vi "Read_LCR_Meter_4192A.vi"() -> ()   [LabVIEW 2018]
panel:
  in  "GPIB addess":string="0:17"
  out "display B":dbl=20.0 format="%.3e"
  out "display A":dbl=0.02 format="%.3e"
  in  "Freq Value (Hz) (25Hz)":dbl=25.0
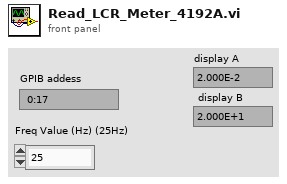
[diagram p1: front panel]
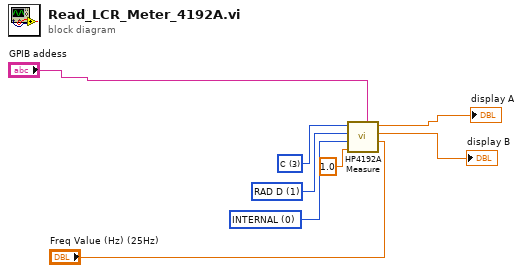
[diagram p0: block diagram]
diagram:
  w2 = i16 1 items=["DEG Q", "RAD D", "         R/G"] ("function B (deg q:0)")
  w3 = i16 3 items=["Z/Y", "R/G", "L", "C"] ("function A (z/y:0)")
  w4 = i16 0 items=["INTERNAL", "EXTERNAL", "HOLD/MANUAL"] ("trigger (internal:0)")
  n1 = call "HP4192A Measure.vi"("OSC level (V)"=1.0, "test signal\nfreq (Hz)"="Freq Value (Hz) (25Hz)", "GPIB addess"="GPIB addess", "trigger (internal:0)"=w4, "function B (deg q:0)"=w2, "function A (z/y:0)"=w3) -> ("display B"=→"display B":dbl, "display A"=→"display A":dbl)  [unwired: 4 in]
